vi "Edit_calibration_coeff_7-04.vi"() -> ()   [LabVIEW 2010]
uses:
  Controls/File_Selector_Type.ctl
  Globals/Meas_global.vi
panel:
  in  "bkgnd Variance":string
  in  "bkgnd":string
  in  "C":string
  in  "Previous Choice":path
  in  "Search String":string
  in  "Boolean":bool
  in  "Pause Mode":enum16{"Continuous Running", "After Each File"}(ring)
  in  "At Dialog Prompt Post Process":T1
  out "Files Processed":i32(slide) scale=0.0..1.0
  in  "stop":bool
  out "Files To Process":path[](array[path])
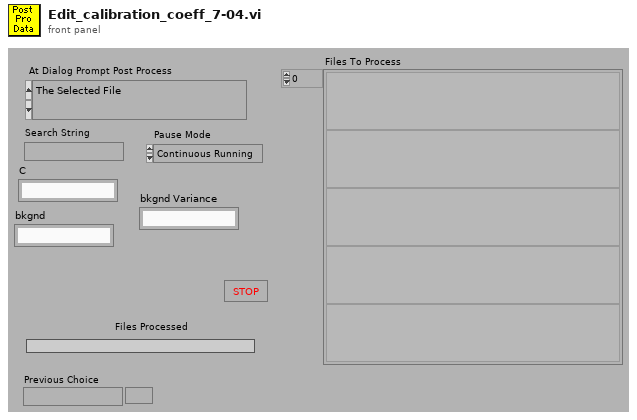
[diagram p1: front panel]
types:
  T1 = typedef "File_Selector_Type.ctl" = enum16{"The Selected File", "The Selected Folder", "Files containing the search string in the selected folder", "All files listed in selected file"}
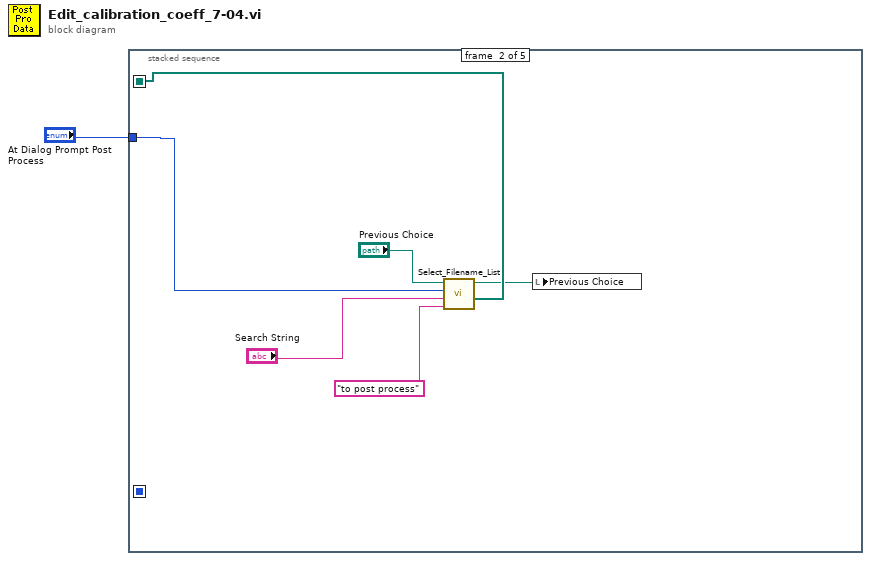
[diagram p0: block diagram]
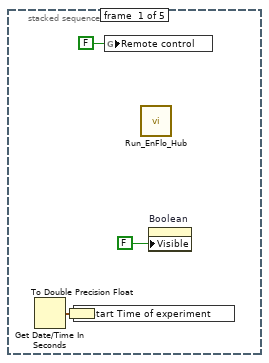
[diagram p2: hidden frame]
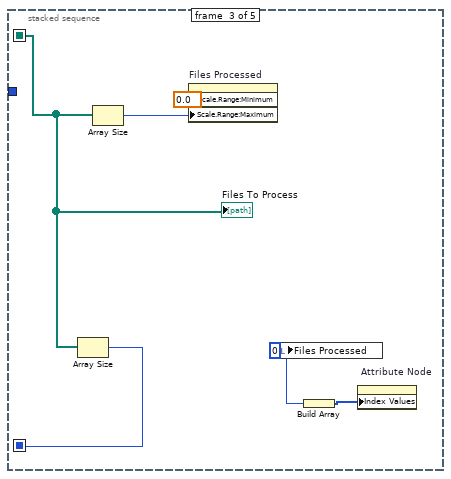
[diagram p3: hidden frame]
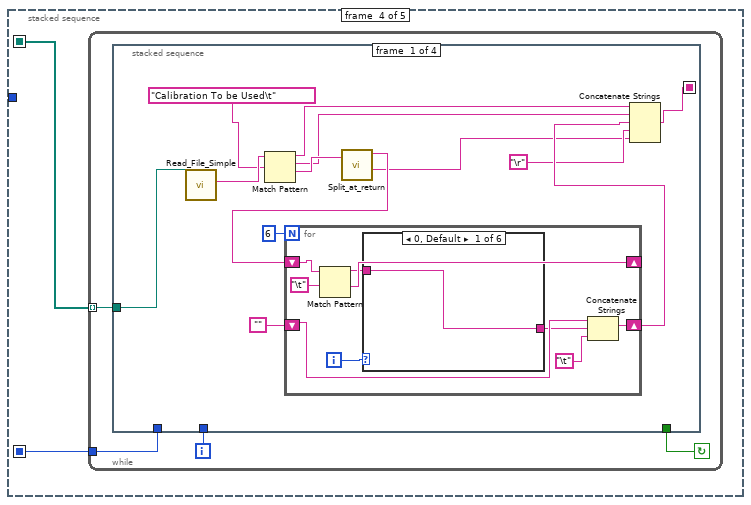
[diagram p4: hidden frame]
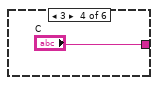
[diagram p7: hidden frame]
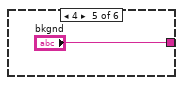
[diagram p8: hidden frame]
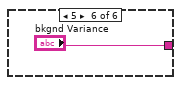
[diagram p9: hidden frame]
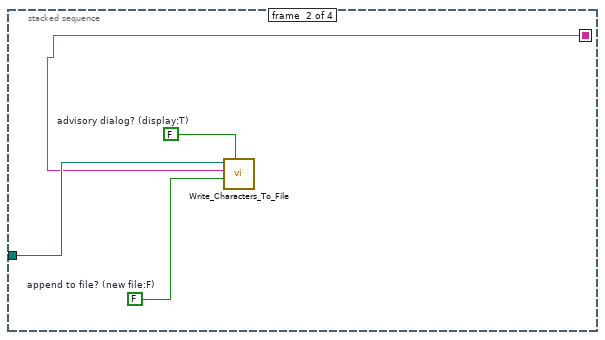
[diagram p10: hidden frame]
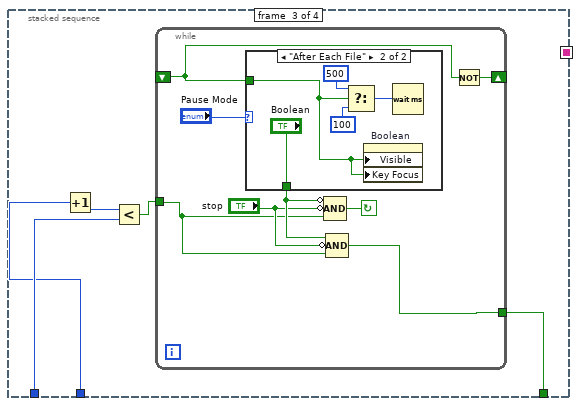
[diagram p11: hidden frame]
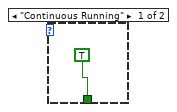
[diagram p12: hidden frame]
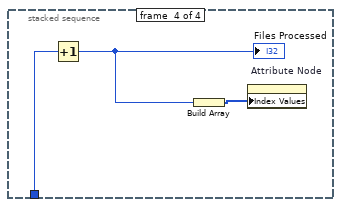
[diagram p13: hidden frame]
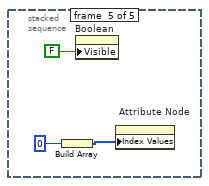
[diagram p14: hidden frame]
diagram:
  n1 = stacked-sequence {
    seq-local: [_ _ w17 _ _] -> [_ _ _ w19 _]
    seq-local: [_ w10 _ _ _] -> [_ _ w12 w18 _]
    tunnel: "At Dialog Prompt Post Process" -> [_ w11 _ _ _]
    frame #0 {
      n2 = Get Date/Time In Seconds() -> (seconds since 1Jan1904=w2:timestamp)
      n3 = To Double Precision Float(number=w2) -> (double precision float=w3:dbl)
      n4 = global write "Meas_global.vi" "Start Time of experiment"(w3) -> ()
      n5 = global write "Meas_global.vi" "Remote control"(FALSE ("Remote control")) -> ()
      n6 = call "Run_EnFlo_Hub.vi"() -> ()  [unwired: 8 in]
      n7 = property on="Boolean" class="Bool"("Visible"=FALSE ("Write Attribute")) -> ()  [unwired: 2 in, 2 out]
    }
    frame #1 {
      n8 = call "Select_Filename_List.vi"("File Type"="to post process", "Search String"="Search String", "At Dialog Prompt Post Process"=w11, "Previous Choice"="Previous Choice") -> ("Selected files"=w10:path[], "Choosen path"=w6:path)  [unwired: 2 in, 1 out]
      n9 = local write "Previous Choice"(w6) -> ()
    }
    frame #2 {
      w13 = 0 ("Files Processed")
      n10 = Array Size(array=w12) -> (size(s)=w17:i32)
      n11 = Array Size(array=w12) -> (size(s)=w15:i32)
      n12 = property on="Files Processed" class="Slide (strict)"("Scale.Range:Minimum"=0.0 ("Write Attribute"), "Scale.Range:Maximum"=w15) -> ()  [unwired: 2 in, 2 out]
      n13 = local write "Files Processed"(w13) -> ()
      n14 = Build Array(w13) -> (w14:i32[])
      n15 = property on="Attribute Node" class="Arr (strict)"("Index Values"=w14) -> ()  [unwired: 2 in, 2 out]
      "Files To Process" <- w12
    }
    frame #3 {
      n16 = while {
        tunnel: w18 -> [w20] mode=indexing
        tunnel: w19 -> [w23]
        i -> [w22]
        stop <- w21 continue-if-true
        n17 = stacked-sequence {
          seq-local: [w26 _ _ _] -> [_ w52 _ _]
          tunnel: w20 -> [w36 w55 _ _]
          tunnel: w23 -> [_ _ w58 _]
          tunnel: w22 -> [_ _ w57 w76]
          tunnel: [_ _ w56 _] -> w21
          frame #0 {
            n18 = call "Read_File_Simple.vi"("Filename"=w36) -> ("string"=w33:string)  [unwired: 4 in, 5 out]
            n19 = Match Pattern(string=w33, regular expression="Calibration To be Used\t" ("Variable name")) -> (before substring=w29:string, match substring=w28:string, after substring=w31:string)  [unwired: 1 in, 1 out]
            n20 = call "Split_at_return.vi"("String"=w31) -> ("before substring"=w30:string, "after substring"=w24:string)  [unwired: 1 in, 2 out]
            n21 = for {
              N: 6 -> [_]
              shift-right: [w39] -> _
              shift-left: w30 -> [w44]
              shift-right: [w40] -> w27
              shift-left: "" -> [w42]
              i -> [w43]
              n22 = Match Pattern(string=w44, regular expression="\t") -> (before substring=w37:string, after substring=w39:string)  [unwired: 1 in, 2 out]
              n23 = case shown="0, Default" w43 {
                tunnel: [w46 w47 w48 "C" "bkgnd" "bkgnd Variance"] -> w38
                tunnel: w37 -> [w46 w47 w48 _ _ _]
                frame 0, Default {
                }
                frame 1 {
                }
                frame 2 {
                }
                frame 3 {
                }
                frame 4 {
                }
                frame 5 {
                }
              }
              n24 = Concatenate Strings(w42, w38, "\t") -> (w40:string)
            }
            n25 = Concatenate Strings(w29, w28, w27, "\r", w24) -> (w26:string)
          }
          frame #1 {
            w53 = FALSE  # append to file? (new file:F)
            w54 = FALSE  # advisory dialog? (display:T)
            n26 = call "Write_Characters_To_File.vi"("file path (dialog if empty)"=w55, "advisory dialog? (display:T)"=w54, "character string"=w52, "append to file? (new file:F)"=w53) -> ()  [unwired: 4 in, 1 out]
          }
          frame #2 {
            n27 = Increment(x=w57) -> (x+1=w60:i32)
            n28 = Less?(x=w60, y=w58) -> (x < y?=w59:bool)
            n29 = while {
              shift-left: _ -> [w66]
              shift-right: [w67] -> _
              tunnel: [w61] -> w56
              tunnel: w59 -> [w62]
              stop <- w65 continue-if-true
              n30 = case shown="\"After Each File\"" "Pause Mode" {
                tunnel: [TRUE "Boolean"] -> w64
                tunnel: w66 -> [_ w73]
                frame "Continuous Running" {
                }
                frame "After Each File" {
                  n31 = Select(t=u32 500 ("milliseconds to wait"), s=w73, f=u32 100) -> (s? t:f=w70:u32)
                  n32 = property on="Boolean" class="Bool"("Visible"=w73, "Key Focus"=w73) -> ()  [unwired: 2 in, 2 out]
                  n33 = Wait (ms)(milliseconds to wait=w70) -> ()  [unwired: 1 out]
                }
              }
              n34 = Compound Arithmetic op=AND(invert w64, invert "stop", w62) -> (w65:bool)
              n35 = Compound Arithmetic op=AND(w64, invert "stop", w62) -> (w61:bool)
              n36 = Not(x=w66) -> (.not. x?=w67:bool)
            }
          }
          frame #3 {
            n37 = Increment(x=w76) -> (x+1=w75:i32)
            "Files Processed" <- w75
            n38 = Build Array(w75) -> (w77:i32[])
            n39 = property on="Attribute Node" class="Arr (strict)"("Index Values"=w77) -> ()  [unwired: 2 in, 2 out]
          }
        }
      }
    }
    frame #4 {
      n40 = Build Array(0) -> (w79:i32[])
      n41 = property on="Boolean" class="Bool"("Visible"=FALSE ("Write Attribute")) -> ()  [unwired: 2 in, 2 out]
      n42 = property on="Attribute Node" class="Arr (strict)"("Index Values"=w79) -> ()  [unwired: 2 in, 2 out]
    }
  }
